vi "Init.vi"(3 "Container State":T5, 4 "Previous State":variant, 5 "Previous Version":T4) -> (2 "Current State":T1={"Prompt"="Click to add", "Listbox"=refnum, "Required"={"Strings"=[], "Bottom"=FALSE, "Italic"=FALSE, "FG"=0, "BG"=0, "Bold"=FALSE}, "Items"=[], "Req'd"=[], "Events"={"Items Changed"=refnum, "List Changed"=refnum}, "Max Rows"=-1, "Default name"=""})   [LabVIEW 2015, in "KListboxEx.xctl"]
uses:
  KListboxEx.xctl
  State.ctl
  Required.ctl
  Events.ctl
  Event Action.ctl
  <vilib>/_xctls/Container State.ctl
  <vilib>/_xctls/Version.ctl
  State V1.ctl
  <vilib>/_xctls/XControlSupport.lvlib
panel:
  in  "Default Indicator State":T1={"Prompt"="Click to add", "Listbox"=refnum, "Required"={"Strings"=[], "Bottom"=FALSE, "Italic"=FALSE, "FG"=0, "BG"=16777215, "Bold"=FALSE}, "Items"=[], "Req'd"=[], "Events"={"Items Changed"=refnum, "List Changed"=refnum}, "Max Rows"=-1, "Default name"=""}
  in  "Default Control State":T1={"Prompt"="Click to add", "Listbox"=refnum, "Required"={"Strings"=[], "Bottom"=FALSE, "Italic"=TRUE, "FG"=0, "BG"=16777215, "Bold"=FALSE}, "Items"=[], "Req'd"=[], "Events"={"Items Changed"=refnum, "List Changed"=refnum}, "Max Rows"=-1, "Default name"=""}
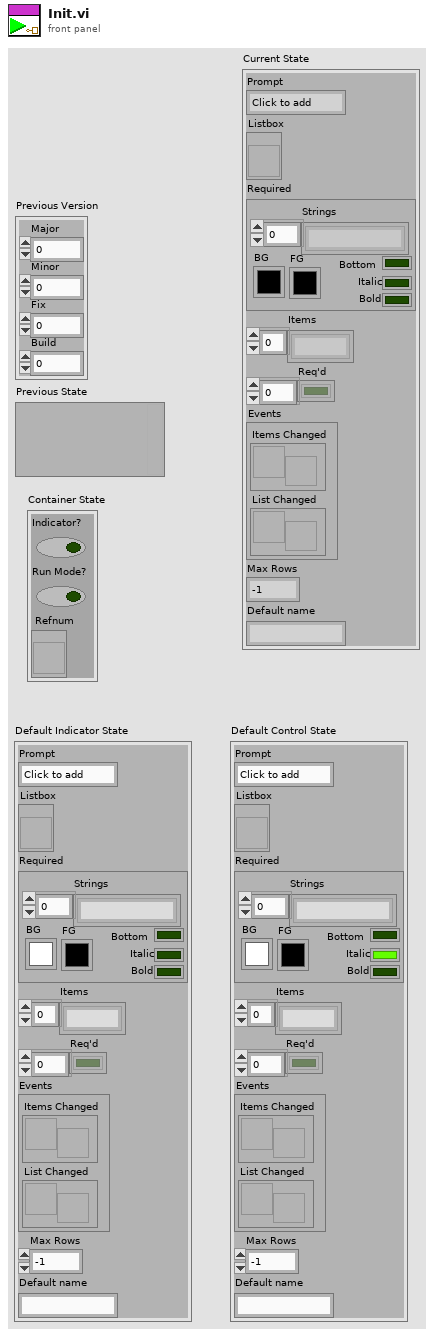
[diagram p1: front panel]
types:
  T1 = typedef "KListboxEx.xctl/State.ctl" = cluster{"Prompt":string, "Listbox":refnum<vi>, "Required":T2, "Items":string[], "Req'd":bool[], "Events":T3, "Max Rows":i32, "Default name":string}
  T2 = typedef "KListboxEx.xctl/Required.ctl" = cluster{"Strings":string[], "Bottom":bool, "Italic":bool, "FG":u32, "BG":u32, "Bold":bool}
  T3 = typedef "KListboxEx.xctl/Events.ctl" = cluster{"Items Changed":refnum<user-event>, "List Changed":refnum<user-event>}
  T4 = typedef "XControlSupport.lvlib/Version.ctl" = cluster{"Major":u16, "Minor":u16, "Fix":u16, "Build":u16}
  T5 = typedef "XControlSupport.lvlib/Container State.ctl" = cluster{"Indicator?":bool, "Run Mode?":bool, " Refnum":refnum<vi>}
  T6 = typedef "KListboxEx.xctl/State V1.ctl" = cluster{"Prompt":string, "Listbox":refnum<vi>, "Required":T2, "Items":string[], "Req'd":bool[], "Events":T3, "Max Rows":i32}
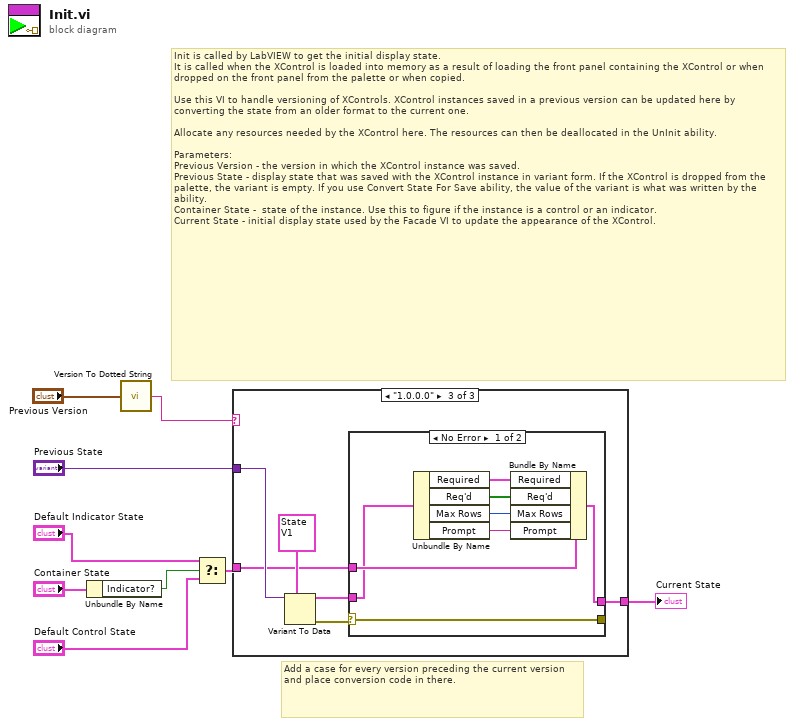
[diagram p0: block diagram]
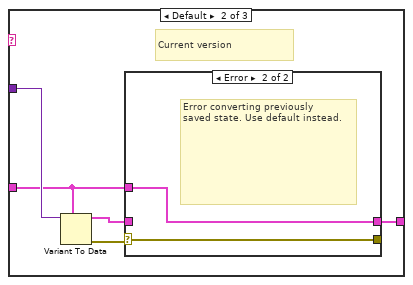
[diagram p3: hidden frame]
diagram:
  # "Add a case for every version preceding the current version and place conversion code in there."
  # "Init is called by LabVIEW to get the initial display state.\nIt is called when the XControl is loaded into memory as a result of loading the front panel containing the XControl or when dropped on the front panel from the palette or when copied.\n\nUse this VI to handle versioning of XControls. XControl instances saved in a previous version can be updated here by converting the state from an older format to the current one.\n\nAllocate any resources needed by the XControl here. The resources can then be deallocated in the UnInit ability.\n\nParameters:\nPrevious Version - the version in which the XControl instance was saved.\nPrevious State - display state that was saved with the XControl instance in variant form. If the XControl is dropped from the palette, the variant is empty. If you use Convert State For Save ability, the value of the variant is what was written by the ability. \nContainer State -  state of the instance. Use this to figure if the instance is a control or an indicator.\nCurrent State - initial display state used by the Facade VI to update the appearance of the XControl."
  n1 = Unbundle By Name("Container State") -> ("Indicator?"=w5:bool)
  n2 = call <vilib>:"Version To Dotted String.vi"("Version"="Previous Version") -> ("String Version"=w2:string)
  n3 = Select(t="Default Indicator State", s=w5, f="Default Control State") -> (s? t:f=w4:T1)
  n4 = case shown="\"1.0.0.0\"" w2 {
    tunnel: "Previous State" -> [_ w15 w25]
    tunnel: [w10 w11 w22] -> w8
    tunnel: w4 -> [w10 w12 w20]
    frame "0.0.0.0" {
      # "Just created, use default state"
    }
    frame Default {
      # "Current version"
      n5 = Variant To Data(type=w12, Variant=w15) -> (data=w13:T1, error out=w14:errorcluster)  [unwired: 1 in]
      n6 = case shown="Error" w14 {
        selector: w14 -> [w17 w18]
        tunnel: w13 -> [w16 _]
        tunnel: [w16 w19] -> w11
        tunnel: w12 -> [_ w19]
        tunnel: [w17 w18] -> _
        frame No Error {
        }
        frame Error {
          # "Error converting previously \nsaved state. Use default instead."
        }
      }
    }
    frame "1.0.0.0" {
      n7 = Variant To Data(type=T6 {"Prompt"="Click to add", "Listbox"=refnum, "Required"={"Strings"=[], "Bottom"=FALSE, "Italic"=FALSE, "FG"=0, "BG"=16777215, "Bold"=FALSE}, "Items"=[], "Req'd"=[], "Events"={"Items Changed"=refnum, "List Changed"=refnum}, "Max Rows"=-1} ("State"), Variant=w25) -> (data=w23:T6, error out=w24:errorcluster)  [unwired: 1 in]
      n8 = case shown="No Error" w24 {
        selector: w24 -> [w33 w35]
        tunnel: w23 -> [w30 _]
        tunnel: [w31 w34] -> w22
        tunnel: [w33 w35] -> _
        tunnel: w20 -> [w32 w34]
        frame No Error {
          n9 = Unbundle By Name(w30) -> ("Required"=w29:T2, "Req'd"=w28:bool[], "Max Rows"=w27:i32, "Prompt"=w26:string)
          n10 = Bundle By Name(cluster=w32, "Required"=w29, "Req'd"=w28, "Max Rows"=w27, "Prompt"=w26) -> (w31:T1)
        }
        frame Error {
          # "Error converting previously \nsaved state. Use default instead."
        }
      }
    }
  }
  "Current State" <- w8
